vi "FGVExample.vi"() -> ()   [LabVIEW 2020]
doc: "Present simple use of FGV with action engine and without. Comments in Polish."
panel:
  out "led":bool
  in  "stop":bool
  out "Chart":dbl(graph)
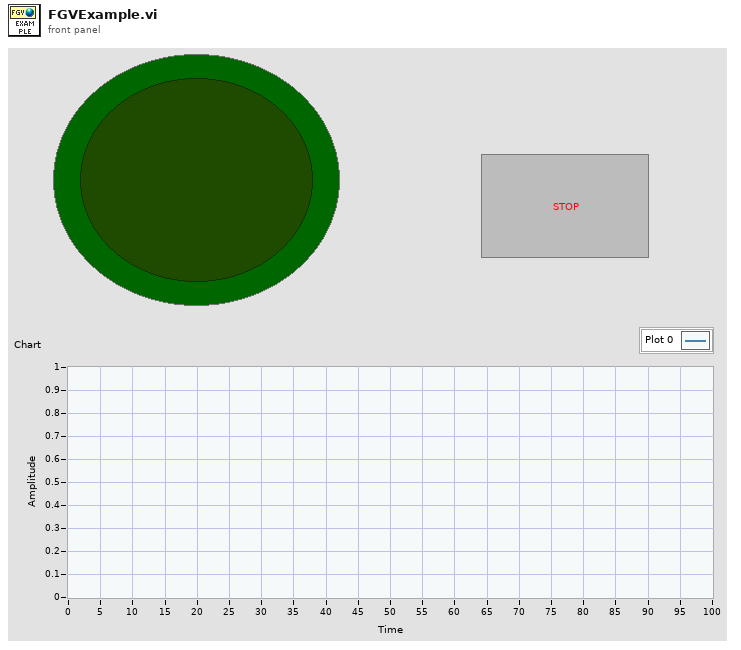
[diagram p1: front panel]
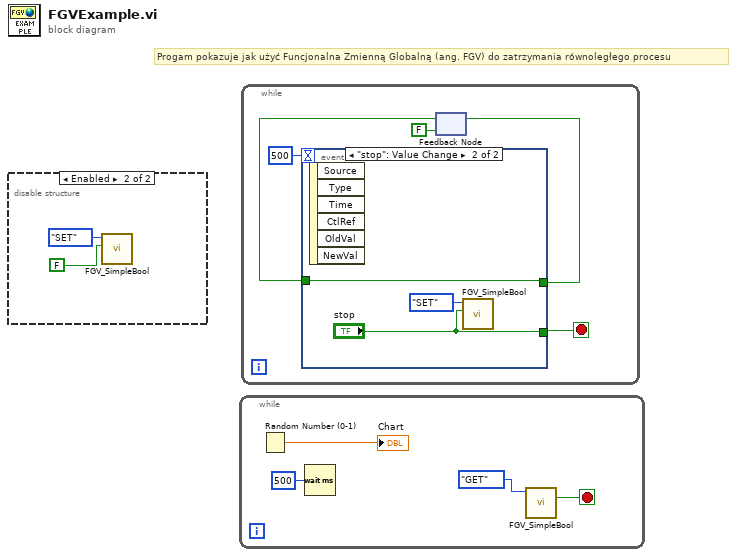
[diagram p0: block diagram]
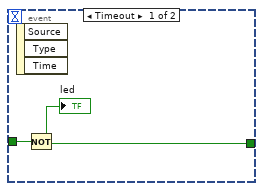
[diagram p3: hidden frame]
diagram:
  # "Progam pokazuje jak użyć Funcjonalna Zmienną Globalną (ang. FGV) do zatrzymania równoległego procesu"
  n1 = disable-structure shown="Enabled" {
    frame Disabled {
    }
    frame Enabled {
      n2 = call "FGV_SimpleBool.vi"("Stop In"=FALSE, "Mode"=enum16{"SET", "GET"}."SET") -> ()  [unwired: 9 in, 1 out]
    }
  }
  n3 = while {
    stop <- w4 stop-if-true
    n4 = Random Number (0-1)() -> (number: 0 to 1=→"Chart":dbl)
    n5 = Wait (ms)(milliseconds to wait=u32 500) -> ()  [unwired: 1 out]
    n6 = call "FGV_SimpleBool.vi"("Mode"=enum16{"SET", "GET"}."GET") -> ("Stop  Out"=w4:bool)  [unwired: 10 in]
  }
  n7 = while {
    stop <- w11 stop-if-true
    n8 = feedback #1(FALSE) -> (w9:bool)
    n9 = event shown="[1] \"stop\": Value Change" {
      selector: _ -> [_ _]
      dyn-events: _ -> [_ _]
      timeout: 500 -> [_ _]
      tunnel: [_ "stop"] -> w11
      tunnel: [w13 w16] -> w10
      tunnel: w9 -> [w12 w16]
      event Timeout {
        n10 = event-data() -> ()  [unwired: 1 in, 3 out]
        n11 = Not(x=w12) -> (.not. x?=w13:bool)
        "led" <- w13
      }
      event "stop": Value Change {
        n12 = event-data() -> ()  [unwired: 1 in, 6 out]
        n13 = call "FGV_SimpleBool.vi"("Stop In"="stop", "Mode"=enum16{"SET", "GET"}."SET") -> ()  [unwired: 9 in, 1 out]
      }
    }
    n14 = feedback-in #1(w10) -> ()
  }
